vi "which_settings_to_load.vi"(8 "error in (no error)":errorcluster, 11 "Which settings to load (in)":cluster{"Boolean":bool, "Setting":string}[](array[cluster])=[{"Boolean"=TRUE, "Setting"="Variables"}, {"Boolean"=TRUE, "Setting"="HSDIO"}, {"Boolean"=TRUE, "Setting"="DAQmx"}, {"Boolean"=TRUE, "Setting"="DDS"}, {"Boolean"=TRUE, "Setting"="Camera"}, {"Boolean"=TRUE, "Setting"="Counters"}, {"Boolean"=TRUE, "Setting"="Filters"}, {"Boolean"=TRUE, "Setting"="AnalogOutput"}, {"Boolean"=TRUE, "Setting"="Notes"}, {"Boolean"=TRUE, "Setting"="GPIB"}, {"Boolean"=TRUE, "Setting"="PhysikInstrumentePiezo"}, {"Boolean"=TRUE, "Setting"="Andor"}] caption="Choose which settings to load:") -> (0 "error out":errorcluster, 3 "Which settings to load":cluster{"Boolean":bool, "Setting":string}[](array[cluster])=[{"Boolean"=TRUE, "Setting"="Variables"}, {"Boolean"=TRUE, "Setting"="HSDIO"}, {"Boolean"=TRUE, "Setting"="DAQmx"}, {"Boolean"=TRUE, "Setting"="DDS"}, {"Boolean"=TRUE, "Setting"="Camera"}, {"Boolean"=TRUE, "Setting"="Counters"}, {"Boolean"=TRUE, "Setting"="Filters"}, {"Boolean"=TRUE, "Setting"="AnalogOutput"}, {"Boolean"=TRUE, "Setting"="Notes"}, {"Boolean"=TRUE, "Setting"="SpectrumAnalyzer"}, {"Boolean"=TRUE, "Setting"="PhysikInstrumentePiezo"}, {"Boolean"=TRUE, "Setting"="Andor"}])   [LabVIEW 2013]
doc: "MTL 2012-12-24\n\nThis VI give allows the user to choose which of the settings will be save into a config file. This allows for flexibility for combining settings from several experiments."
panel:
  in  "Boolean":bool
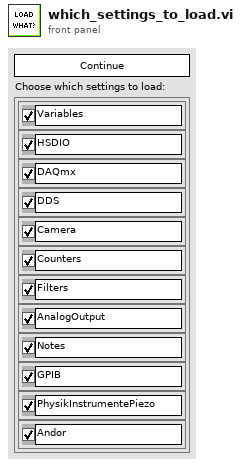
[diagram p1: front panel]
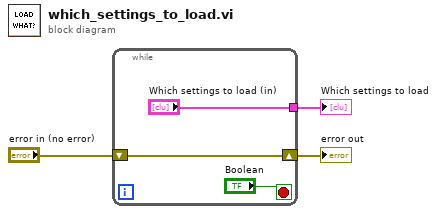
[diagram p0: block diagram]
diagram:
  n1 = while {
    shift-right: [w5] -> w2
    shift-left: "error in (no error)" -> [w5]
    tunnel: ["Which settings to load (in)"] -> w1
    stop <- "Boolean" stop-if-true
  }
  "error out" <- w2
  "Which settings to load" <- w1
